vi "Async Spawn.vi"(9 "Attributes":refnum<class "Attributes.lvclass">, 10 "Unified Actor":refnum<class "Actor.lvclass">) -> (0 "Error out":errorcluster, 2 "Child Attributes":refnum<class "Attributes.lvclass">)   [LabVIEW 2025, in "jettl.lvlib"]
uses:
  jettl.lvlib
  Actor/Actor.lvclass
  Attributes/Attributes/Attributes.lvclass
  Async Actor.vi
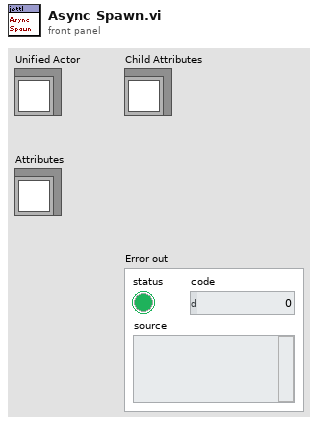
[diagram p1: front panel]
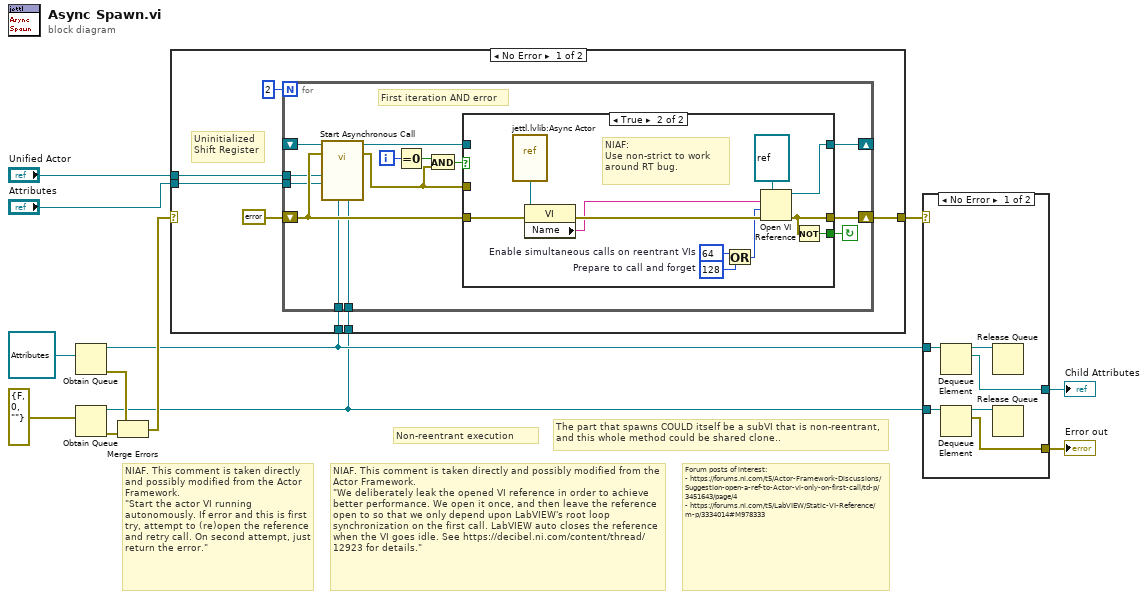
[diagram p0: block diagram]
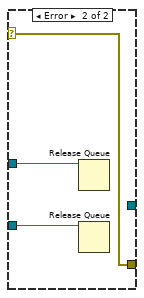
[diagram p2: hidden frame]
diagram:
  # "The part that spawns COULD itself be a subVI that is non-reentrant, and this whole method could be shared clone.."
  # "Forum posts of interest:\n- https://forums.ni.com/t5/Actor-Framework-Discussions/Suggestion-open-a-ref-to-Actor-vi-only-on-first-call/td-p/3451643/page/4\n- https://forums.ni.com/t5/LabVIEW/Static-VI-Reference/m-p/3334014#M978333"
  # "NIAF. This comment is taken directly and possibly modified from the Actor Framework.\n\"We deliberately leak the opened VI reference in order to achieve better performance. We open it once, and then leave the reference open to so that we only depend upon LabVIEW's root loop synchronization on the first call. LabVIEW auto closes the reference when the VI goes idle. See https://decibel.ni.com/content/thread/12923 for details.\""
  # "NIAF. This comment is taken directly and possibly modified from the Actor Framework.\n\"Start the actor VI running autonomously. If error and this is first try, attempt to (re)open the reference and retry call. On second attempt, just return the error.\""
  # "Non-reentrant execution"
  n1 = Obtain Queue(element data type=refnum<class "Attributes.lvclass"> refnum ("jettl.lvlib:Attributes.lvlib:Attributes.lvclass")) -> (queue out=w2:refnum<queue>, error out=w8:errorcluster)  [unwired: 4 in, 1 out]
  n2 = Obtain Queue(element data type=errorcluster {"status"=FALSE, "code"=0, "source"=""} ("Error")) -> (queue out=w1:refnum<queue>, error out=w7:errorcluster)  [unwired: 4 in, 1 out]
  n3 = Merge Errors(w8, w7) -> (w9:errorcluster)
  n4 = case shown="No Error" w9 {
    selector: w9 -> [_ w47]
    tunnel: [w16 w47] -> w12
    tunnel: "Unified Actor" -> [w18 _]
    tunnel: "Attributes" -> [w17 _]
    tunnel: w2 -> [w14 _]
    tunnel: w1 -> [w13 _]
    frame No Error {
      # "Uninitialized\nShift Register"
      n5 = for {
        N: 2 -> [_]
        shift-right: [w33] -> _
        shift-left: _ -> [w32]
        shift-right: [w30] -> w16
        shift-left: errorcluster {"status"=FALSE, "code"=0, "source"=""} ("error out") -> [w26]
        tunnel: w18 -> [w23]
        tunnel: w17 -> [w22]
        tunnel: w14 -> [w21]
        tunnel: w13 -> [w20]
        i -> [w28]
        stop <- w27 continue-if-true
        # "First iteration AND error"
        n6 = call-by-ref "Start Asynchronous Call"(reference=w32, error in=w26, "Queue of Error"=w20, "Queue of Self Attributes"=w21, "Attributes"=w22, "Unified Actor"=w23) -> (reference out=w31:refnum<vi>, error out=w24:errorcluster)  [unwired: 8 in]
        n7 = Equal To 0?(x=w28) -> (x = 0?=w25:bool)
        n8 = And(x=w25, y=w24) -> (x .and. y?=w29:bool)
        n9 = case shown="True" w29 {
          tunnel: [w35 w44] -> w33
          tunnel: [w34 w42] -> w30
          tunnel: w31 -> [w35 _]
          tunnel: w24 -> [w34 _]
          tunnel: [_ w43] -> w27
          tunnel: w26 -> [_ w41]
          frame False {
          }
          frame True {
            w36 = 64  # Enable simultaneous calls on reentrant VIs
            w38 = 128  # Prepare to call and forget
            # "NIAF:\nUse non-strict to work around RT bug."
            n10 = vi-ref "jettl.lvlib:Async Actor.vi"() -> (w40:refnum<vi>)
            n11 = property class="VI"(reference=w40, error in=w41) -> (error out=w46:errorcluster, "Name"=w45:string)  [unwired: 1 out]
            n12 = Or(x=w36, y=w38) -> (x .or. y?=w37:i32)
            n13 = Open VI Reference(type specifier VI Refnum (for type only)=refnum<vi> refnum, vi path=w45, options=w37, error in (no error)=w46) -> (vi reference=w44:refnum<vi>, error out=w42:errorcluster)  [unwired: 2 in]
            n14 = Not(x=w42) -> (.not. x?=w43:bool)
          }
        }
      }
    }
    frame Error {
    }
  }
  n15 = case shown="No Error" w12 {
    selector: w12 -> [_ w54]
    tunnel: w2 -> [w53 w56]
    tunnel: w1 -> [w51 w55]
    tunnel: [w48 w54] -> w5
    tunnel: [w49 _] -> w4
    frame No Error {
      n16 = Dequeue Element(queue=w53) -> (queue out=w52:refnum<queue>, element=w49:refnum<class "Attributes.lvclass">)  [unwired: 2 in, 2 out]
      n17 = Dequeue Element(queue=w51) -> (queue out=w50:refnum<queue>, element=w48:errorcluster)  [unwired: 2 in, 2 out]
      n18 = Release Queue(queue=w52) -> ()  [unwired: 2 in, 3 out]
      n19 = Release Queue(queue=w50) -> ()  [unwired: 2 in, 3 out]
    }
    frame Error {
      n20 = Release Queue(queue=w56) -> ()  [unwired: 2 in, 3 out]
      n21 = Release Queue(queue=w55) -> ()  [unwired: 2 in, 3 out]
    }
  }
  "Error out" <- w5
  "Child Attributes" <- w4
